vi "SEA_TORQUE_CONTROL.vi"() -> ()   [LabVIEW 2019]
uses:
  Torque control target data.ctl
  <vilib>/Platform/TimedLoop/XDataNode/timing_clust.ctl
  <vilib>/Platform/TimedLoop/XDataNode/nitl_modes.ctl
  <vilib>/Platform/TimedLoop/XDataNode/wakeup.ctl
  <vilib>/FPGAPlugInAG/sbRIO-9627/niLvFpga_Open_sbRIO-9627.vi
  <vilib>/rvi/interface/common/dynamic/niFpgaDynamicAddResources.vi
  <vilib>/Utility/error.llb/Error Cluster From Error Code.vi
  <vilib>/rvi/errors/niLvFpgaAdjustHostInterfaceError.vi
  <vilib>/FPGAPlugInAG/Dynamic/niLvFpga_Close_Dynamic.vi
  <vilib>/rvi/interface/nirviOpenFPGA/nirviOpenFPGA.xnode
  FPGA Bitfiles/seafinalexperime_FPGATarget_SEALOWERLEVELCON_meT+vsors+U.lvbitx
  SEA_LOWER_LEVEL_CONTROL.vi
  <vilib>/platform/TimedLoop/XDataNode/XDataNode.xnode
  <vilib>/rvi/interface/nirviReadWriteControl/nirviReadWriteControl.xnode
  <vilib>/rvi/interface/nirviCloseFPGA/nirviCloseFPGA.xnode
  <vilib>/Platform/TimedLoop/XDataNode/XDNodeRunTimeDep.lvlib
  NiFpgaLv.dll
  <vilib>/rvi/interface/Simulation/niFpgaSimulationCallBeginRW.vi
panel:
  in  "Ki":sgl
  in  "Cluster":T1
  in  "Position Reset":bool
  in  "Position Reset joint side":bool
  in  "KpGain":sgl
  out "Finshed late?":u32
  out "Current":cluster{sgl, "Filtered Current(M2)":sgl}(graph)
  out "Torque":cluster{sgl, sgl}(graph)
  in  "stop":bool
  out "control_ip":sgl
  out "motor direction":bool
  in  "lower limit":sgl
  in  "upper limit":sgl
  in  "Kp":sgl
  in  "Amplitude":sgl
  in  "frequency":sgl
  in  "Current Offset":sgl
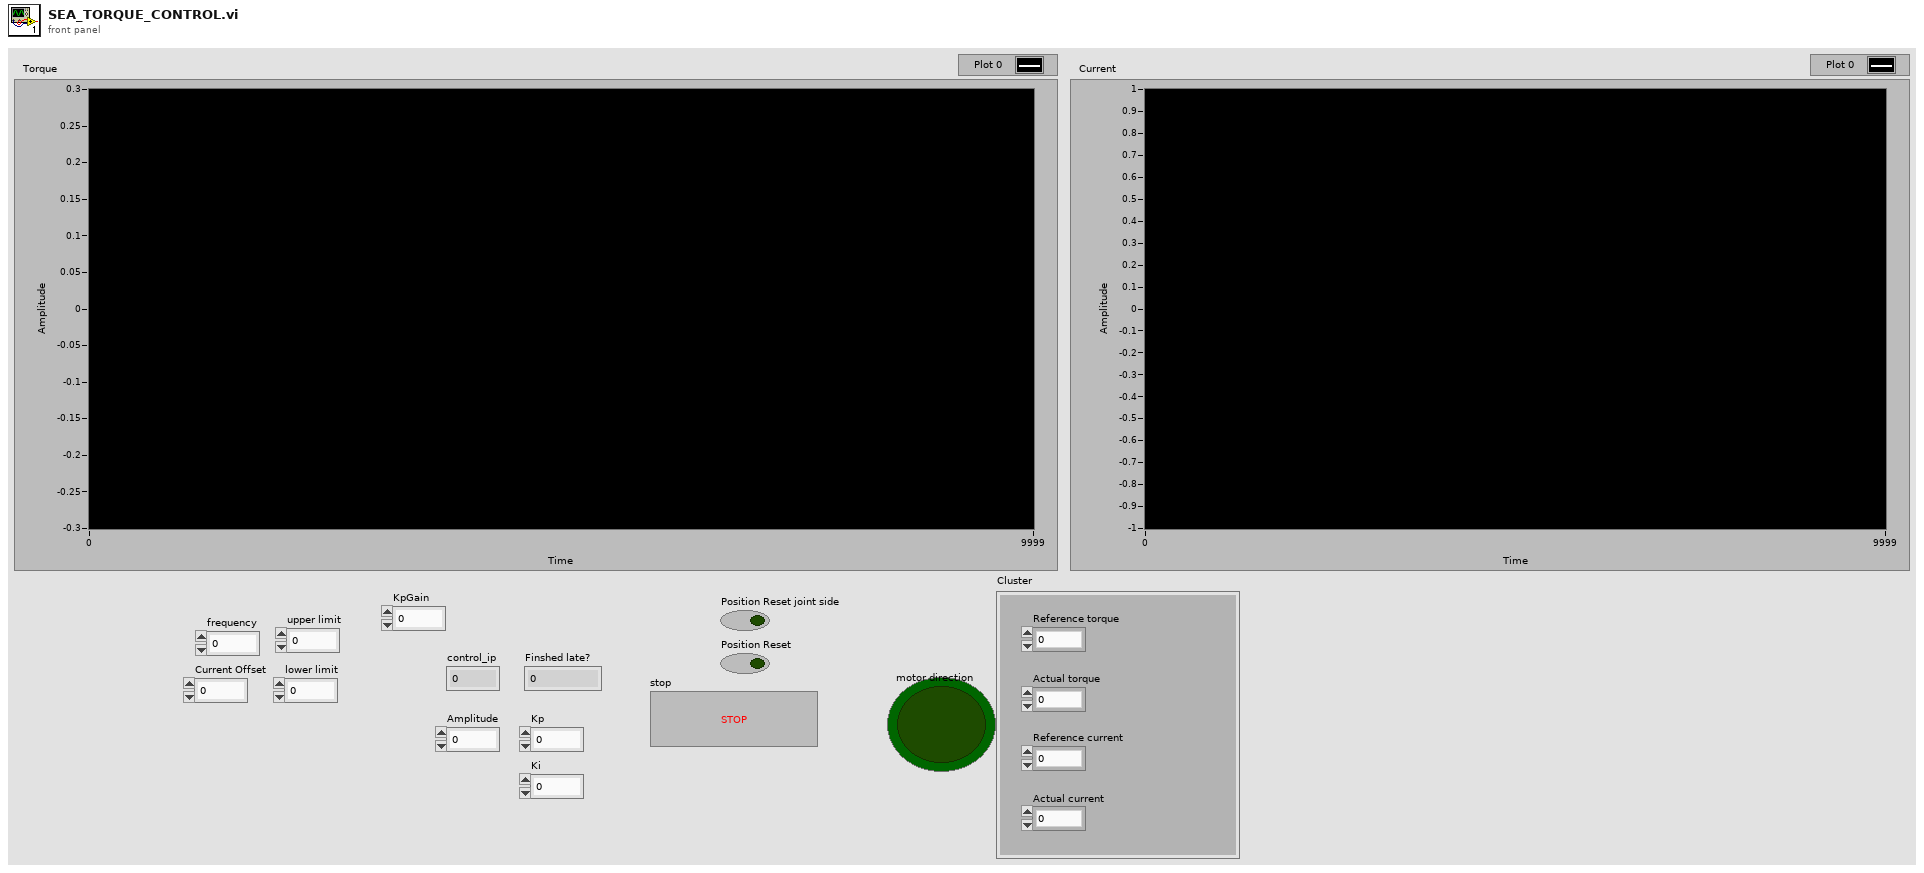
[diagram p1: front panel]
types:
  T1 = typedef "Torque control target data.ctl" = cluster{"Reference torque":sgl, "Actual torque":sgl, "Reference current":sgl, "Actual current":sgl}
  T2 = typedef "XDNodeRunTimeDep.lvlib/timing_clust.ctl" = cluster{"Expected End [f-1]":u64, "Actual End [f-1]":u64, "Finished Late? [f-1]":bool, "Expected End [i-1]":u64, "Actual End [i-1]":u64, "Finished Late? [i-1]":bool, "Expected Start [i]":u64, "Actual Start [i]":u64, "Expected Start [f]":u64, "Actual Start [f]":u64, "Source Name":string, "Structure Name":string, "Period":i64, "Deadline":i64, "Offset":i64, "Start":i64, "Priority":i32, "Timeout":i32, "Mode":T3, "Wakeup Reason":T4, "Error":errorcluster, "Source Type":string, "Secondary Source Type":string, "Global End Time":u64, "Global Start Time":u64, "Frame Duration":u64, "Iteration Duration":u64, "Assigned CPU":i32, "I/O Scan Engine Mode":u32}
  T3 = typedef "XDNodeRunTimeDep.lvlib/nitl_modes.ctl" = enum32{"No Change", "Process missed periods, maintain original phase", "Discard missed periods, maintain original phase", "Process missed periods, ignore original phase", "Discard missed periods, ignore original phase"}
  T4 = typedef "XDNodeRunTimeDep.lvlib/wakeup.ctl" = enum32{"Normal", "Aborted", "Asynchronous wakeup", "Timing source error", "Timed loop error", "Timeout"}
  T5 = enum16{"open", "open or create", "create or replace", "create", "open (read-only)"}
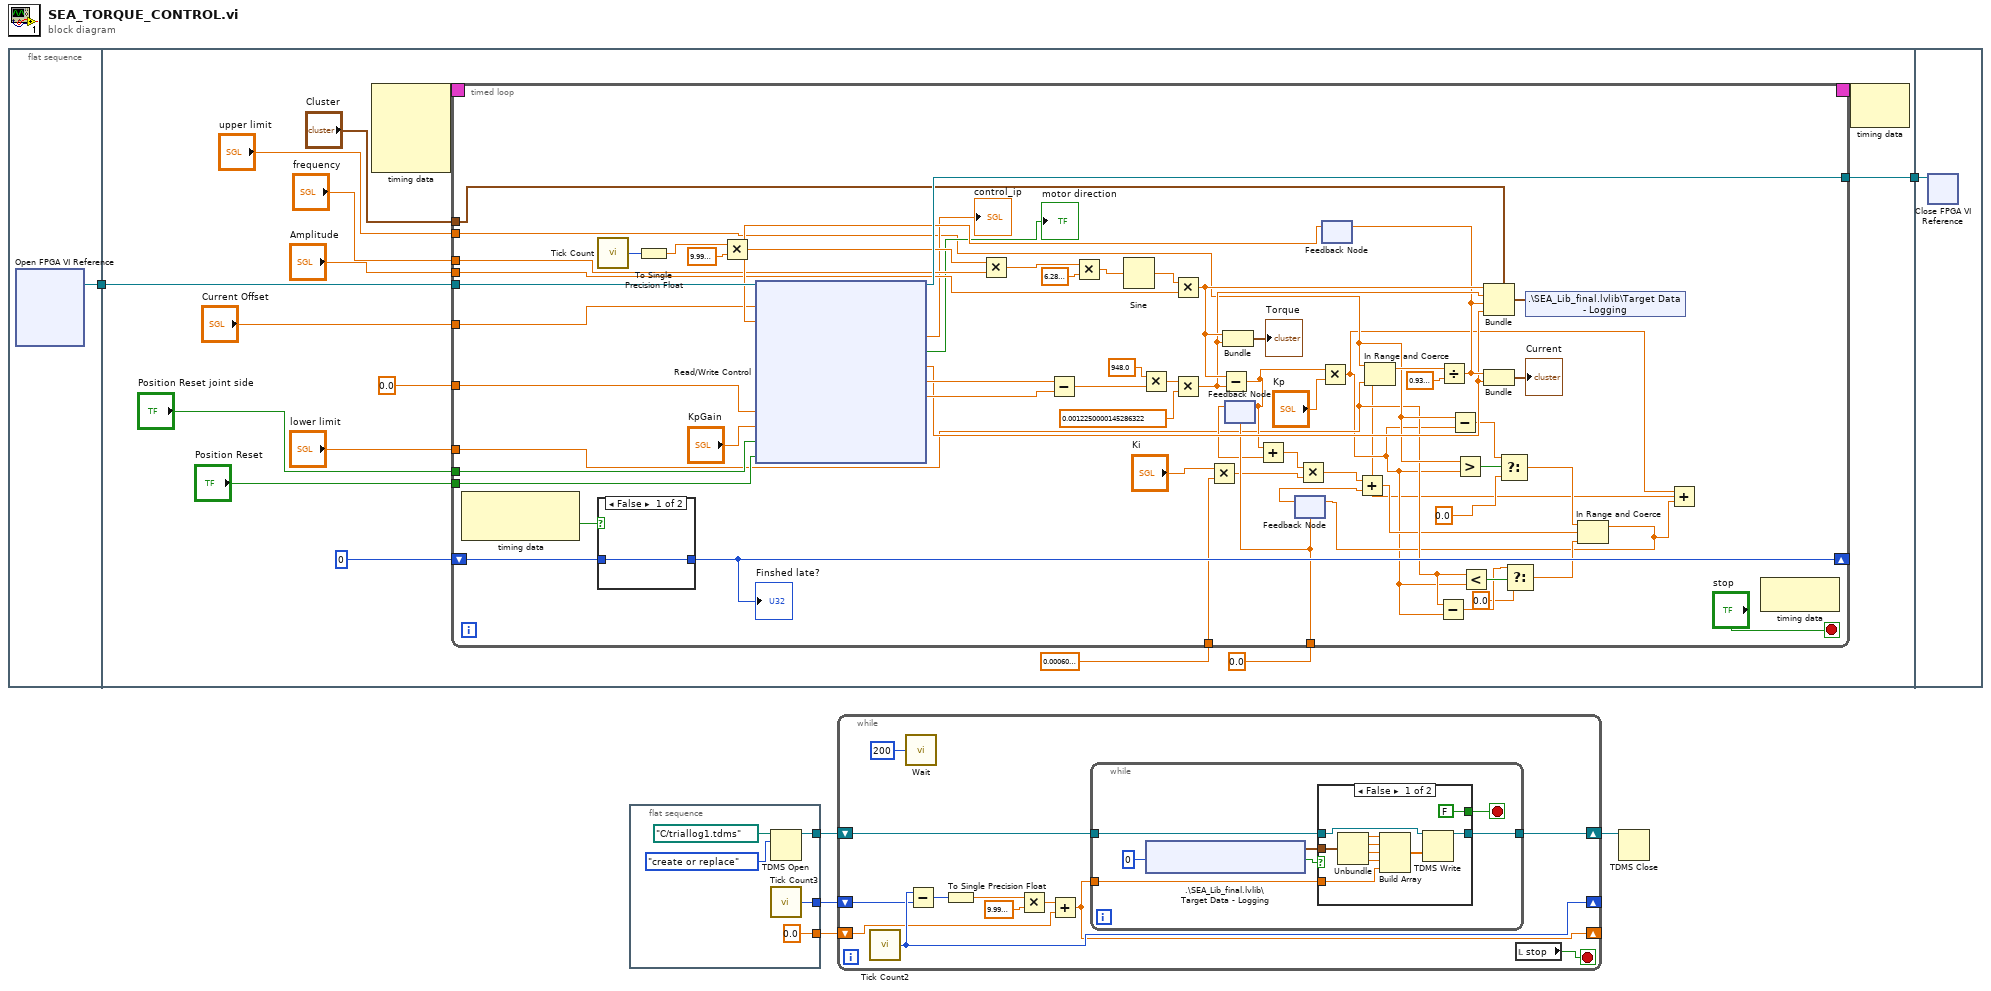
[diagram p0: block diagram]
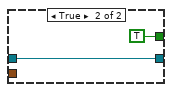
[diagram p2: hidden frame]
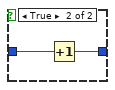
[diagram p3: hidden frame]
diagram:
  n1 = flat-sequence {
    tunnel: [w7] -> w6
    tunnel: w6 -> [w23]
    tunnel: [w22] -> w5
    tunnel: w5 -> [w96]
    frame #0 {
      n2 = xnode "Open FPGA VI Reference"() -> ("FPGA VI Reference Out"=w7:refnum<k20>)  [unwired: 2 in, 1 out]
    }
    frame #1 {
      n3 = node-c288() -> (w21:T2)  [unwired: 4 in]
      n4 = timed-loop {
        tunnel: w23 -> [w87]
        tunnel: [w79] -> w22
        timing: w21 -> [_]
        timing-out: [_] -> w20
        shift-right: [w48] -> _
        shift-left: u32 0 -> [w66]
        tunnel: "Position Reset" -> [w60]
        tunnel: "Position Reset joint side" -> [w59]
        tunnel: "Current Offset" -> [w58]
        tunnel: "frequency" -> [w57]
        tunnel: "Amplitude" -> [w56]
        tunnel: "upper limit" -> [w37]
        tunnel: "lower limit" -> [w32]
        tunnel: "Cluster" -> [w55]
        tunnel: sgl 0.0 -> [w44]
        tunnel: sgl 0.0 ("Tracking zero offset") -> [w47]
        tunnel: sgl 0.0006 ("y") -> [w45]
        stop <- "stop" stop-if-true
        n5 = node-c288() -> (w67:bool)  [unwired: 1 in, 1 out]
        n6 = call "Tick Count"() -> ("Tick Count(uSec)"=w72:u32)
        n7 = case shown="False" w67 {
          tunnel: w66 -> [w88 w90]
          tunnel: [w88 w89] -> w48
          frame False {
          }
          frame True {
            n8 = Increment(x=w90) -> (x+1=w89:u32)
          }
        }
        "Finshed late?" <- w48
        n9 = To Single Precision Float(number=w72) -> (single precision float=w71:sgl)
        n10 = Multiply(x=w71, y=sgl 1e-06) -> (x*y=w69:sgl)
        n11 = Multiply(x=w69, y=w57) -> (x*y=w84:sgl)
        n12 = Multiply(x=w84, y=sgl 6.28) -> (x*y=w83:sgl)
        n13 = Sine(x=w83) -> (sin(x)=w82:sgl)
        n14 = Multiply(x=w82, y=w56) -> (x*y=w65:sgl)
        n15 = Multiply(x="Ki", y=w45) -> (x*y=w40:sgl)
        n16 = feedback #1(w44) -> (w42:sgl)
        n17 = feedback #2(w44) -> (w38:sgl)
        n18 = feedback #3() -> (w77:sgl)  [unwired: 1 in]
        n19 = xnode "Read/Write Control"("FPGA VI Reference In"=w87, "Current Offset"=w58, "reference"=w77, "Tracking zero offset"=w47, "KpGain"="KpGain", "Position Reset joint side"=w59, "Position Reset"=w60) -> ("FPGA VI Reference Out"=w79:refnum<k20>, "control_ip"=→"control_ip":sgl, "motor direction"=→"motor direction":bool, "Filtered Current(M2)"=w62:sgl, "Position(Radians) motor side"=w76:sgl, "Position(Radians) joint side"=w75:sgl)  [unwired: 1 in, 1 out]
        n20 = Subtract(x=w76, y=w75) -> (x-y=w86:sgl)
        n21 = Multiply(x=sgl 948.0, y=w86) -> (x*y=w85:sgl)
        n22 = Multiply(x=w85, y=sgl 0.001225) -> (x*y=w64:sgl)
        n23 = Subtract(x=w65, y=w64) -> (x-y=w43:sgl)
        n24 = Bundle(w65, w64) -> (→"Torque":cluster{sgl, sgl})  [unwired: 1 in]
        n25 = feedback-in #1(w43) -> ()
        n26 = Add(x=w43, y=w42) -> (x+y=w41:sgl)
        n27 = Multiply(x=w41, y=w40) -> (x*y=w39:sgl)
        n28 = Multiply(x=w43, y="Kp") -> (x*y=w25:sgl)
        n29 = Add(x=w39, y=w38) -> (x+y=w29:sgl)
        n30 = Subtract(x=w32, y=w25) -> (x-y=w31:sgl)
        n31 = Subtract(x=w37, y=w25) -> (x-y=w35:sgl)
        n32 = Greater?(x=w37, y=w25) -> (0:w36:bool)
        n33 = Less?(x=w32, y=w25) -> (x < y?=w33:bool)
        n34 = Select(t=w35, s=w36, f=sgl 0.0) -> (s? t:f=w28:sgl)
        n35 = Select(t=w31, s=w33, f=sgl 0.0) -> (s? t:f=w27:sgl)
        n36 = In Range and Coerce(upper limit=w28, x=w29, lower limit=w27) -> (coerced(x)=w26:sgl)  [unwired: 1 out]
        n37 = feedback-in #2(w26) -> ()
        n38 = Add(x=w25, y=w26) -> (x+y=w24:sgl)
        n39 = In Range and Coerce(upper limit=w37, x=w24, lower limit=w32) -> (coerced(x)=w81:sgl)  [unwired: 1 out]
        n40 = Divide(x=w81, y=sgl 0.94) -> (x/y=w63:sgl)
        n41 = feedback-in #3(w63) -> ()
        n42 = Bundle(cluster=w55, "Reference torque"=w65, "Actual torque"=w64, "Reference current"=w63, "Actual current"=w62) -> (w61:T1)
        n43 = Bundle(w63, "Filtered Current(M2)"=w62) -> (→"Current":cluster{sgl, "Filtered Current(M2)":sgl})  [unwired: 1 in]
        n44 = shared-variable ".\\SEA_Lib_final.lvlib\\Target Data - Logging"(w61) -> ()  [unwired: 1 in, 1 out]
        n45 = node-c288() -> ()  [unwired: 1 in, 1 out]
      }
      n46 = node-c288(w20) -> ()  [unwired: 1 out]
    }
    frame #2 {
      n47 = xnode "Close FPGA VI Reference"("FPGA VI Reference In"=w96) -> ()  [unwired: 1 in, 1 out]
    }
  }
  n48 = flat-sequence {
    tunnel: [w99] -> w4
    tunnel: [w98] -> w2
    tunnel: [sgl 0.0] -> w1
    frame #0 {
      n49 = TDMS Open(10:T5."create or replace" ("operation (0:open)"), 11:path "C:/triallog1.tdms" ("file path")) -> (3:w99:refnum<k34>)  [unwired: 5 in, 1 out]
      n50 = call "Tick Count3"() -> ("Tick Count(uSec)"=w98:u32)
    }
  }
  n51 = while {
    shift-right: [w111] -> w3
    shift-left: w4 -> [w113]
    shift-right: [w109] -> _
    shift-left: w2 -> [w108]
    shift-right: [w102] -> _
    shift-left: w1 -> [w103]
    stop <- w112 stop-if-true
    n52 = call "Tick Count2"() -> ("Tick Count(uSec)"=w109:u32)
    n53 = call "Wait"("Count(uSec)"=u32 200) -> ()  [unwired: 1 out]
    n54 = Subtract(x=w109, y=w108) -> (x-y=w107:u32)
    n55 = To Single Precision Float(number=w107) -> (single precision float=w106:sgl)
    n56 = Multiply(x=w106, y=sgl 1e-06) -> (x*y=w105:sgl)
    n57 = Add(x=w105, y=w103) -> (x+y=w102:sgl)
    n58 = while {
      tunnel: w113 -> [w117]
      tunnel: [w115] -> w111
      tunnel: w102 -> [w114]
      stop <- w118 stop-if-true
      n59 = shared-variable ".\\SEA_Lib_final.lvlib\\Target Data - Logging"(0 ("ms timeout (0)")) -> (w116:T1, w119:bool)  [unwired: 1 in, 1 out]
      n60 = case shown="False" w119 {
        tunnel: [FALSE TRUE] -> w118
        tunnel: w117 -> [w130 w131]
        tunnel: w116 -> [w129 _]
        tunnel: [w123 w131] -> w115
        tunnel: w114 -> [w121 _]
        frame False {
          n61 = Unbundle(w129) -> ("Reference torque"=w128:sgl, "Actual torque"=w127:sgl, "Reference current"=w126:sgl, "Actual current"=w125:sgl)
          n62 = Build Array(w128, w127, w126, w125, w121) -> (w124:sgl[])
          n63 = TDMS Write(0:w130, 9:w124) -> (4:w123:refnum<k34>)  [unwired: 4 in, 3 out]
        }
        frame True {
        }
      }
    }
    n64 = local read "stop"() -> (w112:bool)
  }
  n65 = TDMS Close(11:w3) -> ()  [unwired: 1 in, 2 out]
